vi "NewportMotorStopped.vi"(8 "error in (no error)":errorcluster, 9 "Channel":i32, 10 "Controller #":string, 11 "VISA Refnum in":refnum<visa-resource-name>) -> (0 "error out":errorcluster)   [LabVIEW 2014]
panel:
  out "Response 2":string
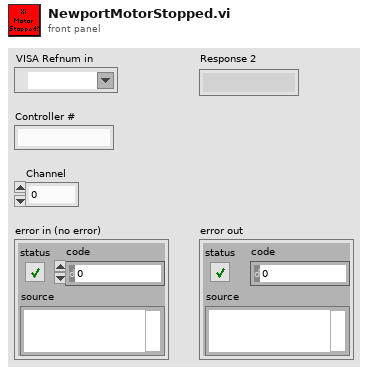
[diagram p1: front panel]
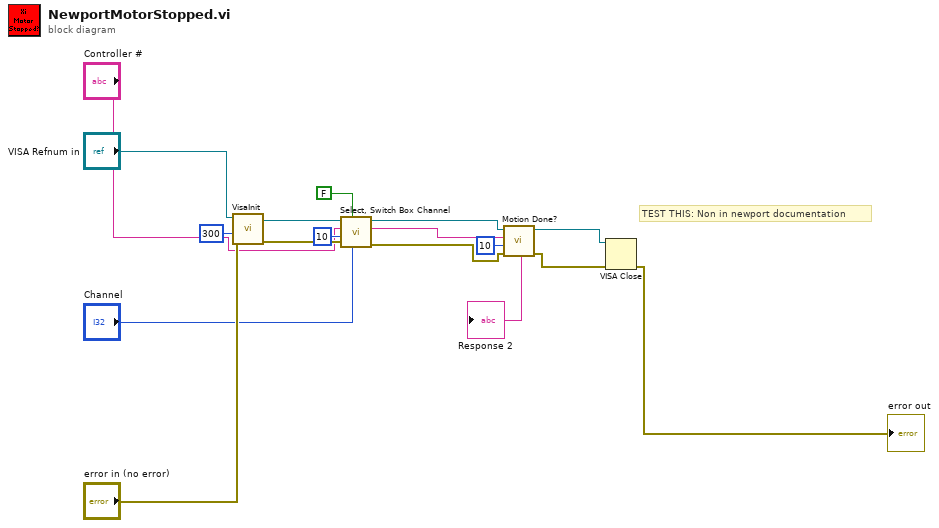
[diagram p0: block diagram]
diagram:
  # "TEST THIS: Non in newport documentation"
  n1 = call <userlib>:"VisaInit.vi"("error in (no error)"="error in (no error)", "Timeout (ms)"=u32 300, "Visa Session"="VISA Refnum in") -> ("error out"=w6:errorcluster, "Visa Handle"=w5:refnum<visa-resource-name>)  [unwired: 4 in]
  n2 = call <userlib>:"Select, Switch Box Channel.vi"("Value"="Channel", "Query?"=FALSE, "error in (no error)"=w6, "Delay (ms)"=u32 10, "Controller #"="Controller #", "VISA Handle"=w5) -> ("error out"=w12:errorcluster, "Dup Controller #"=w14:string, "Dup VISA Handle"=w13:refnum<visa-resource-name>)  [unwired: 2 out]
  n3 = call <userlib>:"Motion Done?.vi"("error in (no error)"=w12, "Delay (ms)"=u32 10, "Controller #"=w14, "VISA Handle"=w13) -> ("error out"=w16:errorcluster, "Response"=→"Response 2":string, "Dup VISA Handle"=w15:refnum<visa-resource-name>)  [unwired: 1 in, 2 out]
  n4 = VISA Close(VISA resource name=w15, error in (no error)=w16) -> (error out=→"error out":errorcluster)
